vi "GetNextIndex.vi"(10 "Data":variant[][](array[variant]), 11 "Column":i32) -> (3 "NextIndex":i32)   [LabVIEW 2018]
doc: "Given the column number where the table index is kept, find the last index and increment it.\n\nCopyright © 2011 Epimedia, Inc. All Rights Reserved.\n\nThe Epimedia Application Library is Copyright © 2009-2011 Epimedia, Inc. \nAll Rights Reserved. Used under license."
panel:
  out "ErrorOut":errorcluster
  in  "ErrorIn":errorcluster
  # "Copyright © 2011 Epimedia, Inc. All Rights Reserved.\n\nThe Epimedia Application Library is Copyright © 2009-2011 Epimedia, Inc. \nAll Rights Reserved. Used under license."
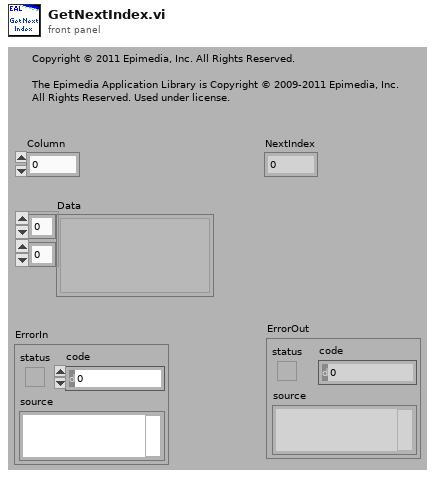
[diagram p1: front panel]
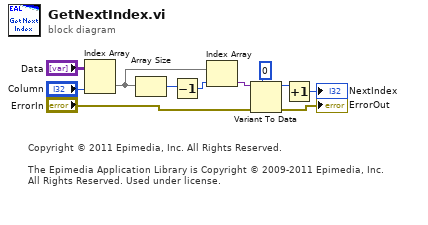
[diagram p0: block diagram]
diagram:
  # "Copyright © 2011 Epimedia, Inc. All Rights Reserved.\n\nThe Epimedia Application Library is Copyright © 2009-2011 Epimedia, Inc. \nAll Rights Reserved. Used under license."
  n1 = Index Array(array="Data", index (col)="Column") -> (element=w5:variant[])  [unwired: 1 in]
  n2 = Array Size(array=w5) -> (size(s)=w6:i32)
  n3 = Decrement(x=w6) -> (x-1=w7:i32)
  n4 = Index Array(array=w5, index=w7) -> (element=w8:variant)
  n5 = Variant To Data(error in="ErrorIn", type=0 ("disabled index (col)"), Variant=w8) -> (data=w10:i32, error out=→"ErrorOut":errorcluster)
  n6 = Increment(x=w10) -> (x+1=→"NextIndex":i32)
